vi "Write All Results.vi"(10 "Test Passed":bool[](array[boolean]), 11 "Test Class.lvclass":refnum<class "Test Class.lvclass">) -> ()   [LabVIEW 2017, in "Test Class.lvclass"]
uses:
  Test Class.lvclass
  <vilib>/TSS/ACRObat Test Framework/Core Launcher/Core Manager Methods -- Enum.ctl
  Classes/Application/Class/Application.lvclass
  <vilib>/TSS/ACRObat Test Framework/Core Launcher/Core Launcher.lvlib
  <vilib>/TSS/ACRObat Test Framework/Classes/Data/Data Repo/Class/Data Repo.lvclass
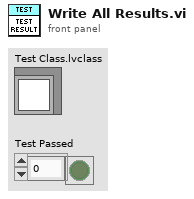
[diagram p1: front panel]
types:
  T1 = typedef "Core Launcher.lvlib/Core Manager Methods -- Enum.ctl" = enum16{"Spawn Objects", "Get Objects", "Destroy Objects"}
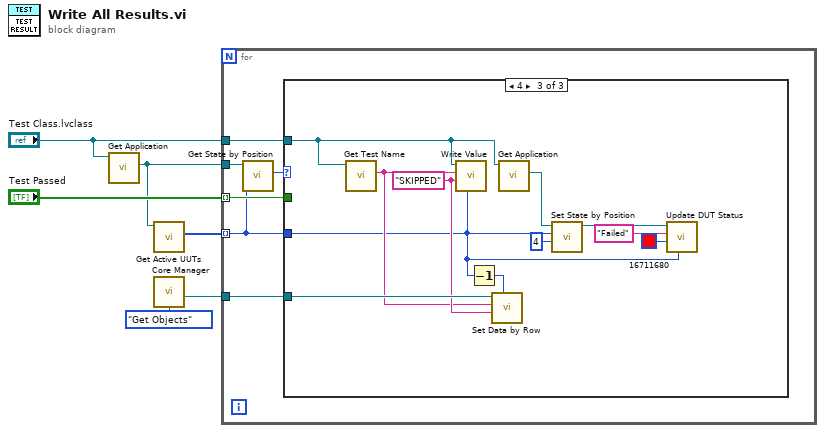
[diagram p0: block diagram]
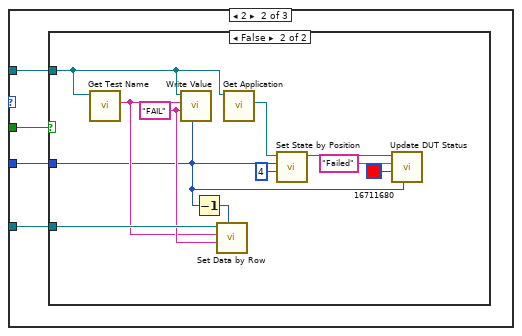
[diagram p3: hidden frame]
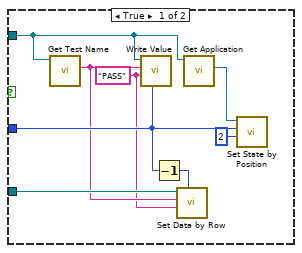
[diagram p4: hidden frame]
diagram:
  n1 = call "Get Application.vi"("Test Class in"="Test Class.lvclass") -> ("Application.lvlib:Application.lvclass"=w1:refnum<class "Application.lvclass">)  [unwired: 9 in, 1 out]
  n2 = call "Get Active UUTs.vi"("Application in"=w1) -> ("Active Positions"=w2:u32[])  [unwired: 8 in, 2 out]
  n3 = call <vilib>:"Core Manager.vi"("Method"=Core_Manager_Methods_--_Enum."Get Objects") -> ("Data Repo"=w4:refnum<class "Data Repo.lvclass">)  [unwired: 6 in, 4 out]
  n4 = for {
    tunnel: "Test Passed" -> [w12] mode=indexing
    tunnel: w4 -> [w11]
    tunnel: "Test Class.lvclass" -> [w10]
    tunnel: w2 -> [w8] mode=indexing
    tunnel: w1 -> [w9]
    n5 = call-dynamic "Get State by Position.vi"("Position"=w8, "Application in"=w9) -> ("State"=w7:u32)  [unwired: 7 in, 2 out]
    n6 = case shown="4" w7 {
      tunnel: w12 -> [_ w16 _]
      tunnel: w8 -> [_ w15 w36]
      tunnel: w10 -> [_ w14 w37]
      tunnel: w11 -> [_ w13 w46]
      frame Default {
      }
      frame 2 {
        n7 = case shown="False" w16 {
          tunnel: w15 -> [w21 w25]
          tunnel: w14 -> [w17 w26]
          tunnel: w13 -> [w22 w30]
          frame True {
            w18 = "PASS" ("Message")
            n8 = call "Get Test Name.vi"("Test Class in"=w17) -> ("Test Name"=w19:string)  [unwired: 9 in, 1 out]
            n9 = call "Write Value.vi"("Position"=w21, "Value"=w18, "Label"=w19, "Test Class in"=w17) -> ()  [unwired: 7 in, 1 out]
            n10 = Decrement(x=w21) -> (x-1=w20:u32)
            n11 = call <vilib>:"Set Data by Row.vi"("Row"=w20, "Value"=w18, "Header"=w19, "Acrobat Template in"=w22) -> ()  [unwired: 6 in, 2 out]
            n12 = call "Get Application.vi"("Test Class in"=w17) -> ("Application.lvlib:Application.lvclass"=w24:refnum<class "Application.lvclass">)  [unwired: 9 in, 1 out]
            n13 = call-dynamic "Set State by Position.vi"("State"=u32 2, "Position"=w21, "Application in"=w24) -> ()  [unwired: 7 in, 2 out]
          }
          frame False {
            w28 = "FAIL" ("Message")
            n14 = call "Get Test Name.vi"("Test Class in"=w26) -> ("Test Name"=w27:string)  [unwired: 9 in, 1 out]
            n15 = call "Write Value.vi"("Position"=w25, "Value"=w28, "Label"=w27, "Test Class in"=w26) -> ()  [unwired: 7 in, 1 out]
            n16 = Decrement(x=w25) -> (x-1=w29:u32)
            n17 = call <vilib>:"Set Data by Row.vi"("Row"=w29, "Value"=w28, "Header"=w27, "Acrobat Template in"=w30) -> ()  [unwired: 6 in, 2 out]
            n18 = call "Get Application.vi"("Test Class in"=w26) -> ("Application.lvlib:Application.lvclass"=w35:refnum<class "Application.lvclass">)  [unwired: 9 in, 1 out]
            n19 = call-dynamic "Set State by Position.vi"("State"=u32 4, "Position"=w25, "Application in"=w35) -> ("Application out"=w33:refnum<class "Application.lvclass">)  [unwired: 7 in, 1 out]
            n20 = call "Update DUT Status.vi"("Position"=w25, "BG Color"=u32 16711680, "Message ('')"="Failed", "Application in"=w33) -> ()  [unwired: 6 in, 2 out]
          }
        }
      }
      frame 4 {
        w39 = "SKIPPED" ("Message")
        n21 = call "Get Test Name.vi"("Test Class in"=w37) -> ("Test Name"=w38:string)  [unwired: 9 in, 1 out]
        n22 = call "Write Value.vi"("Position"=w36, "Value"=w39, "Label"=w38, "Test Class in"=w37) -> ()  [unwired: 7 in, 1 out]
        n23 = Decrement(x=w36) -> (x-1=w40:u32)
        n24 = call <vilib>:"Set Data by Row.vi"("Row"=w40, "Value"=w39, "Header"=w38, "Acrobat Template in"=w46) -> ()  [unwired: 6 in, 2 out]
        n25 = call "Get Application.vi"("Test Class in"=w37) -> ("Application.lvlib:Application.lvclass"=w45:refnum<class "Application.lvclass">)  [unwired: 9 in, 1 out]
        n26 = call-dynamic "Set State by Position.vi"("State"=u32 4, "Position"=w36, "Application in"=w45) -> ("Application out"=w43:refnum<class "Application.lvclass">)  [unwired: 7 in, 1 out]
        n27 = call "Update DUT Status.vi"("Position"=w36, "BG Color"=u32 16711680, "Message ('')"="Failed", "Application in"=w43) -> ()  [unwired: 6 in, 2 out]
      }
    }
  }
